vi "Write Name.vi"(8 "error in (no error)":errorcluster, 10 "Name":string, 11 "Config in":refnum<class "Config.lvclass">) -> (0 "error out":errorcluster, 3 "Config out":refnum<class "Config.lvclass">)   [LabVIEW 2018, in "Config.lvclass"]
uses:
  Config.lvclass
  Config.lvclass/Config.ctl
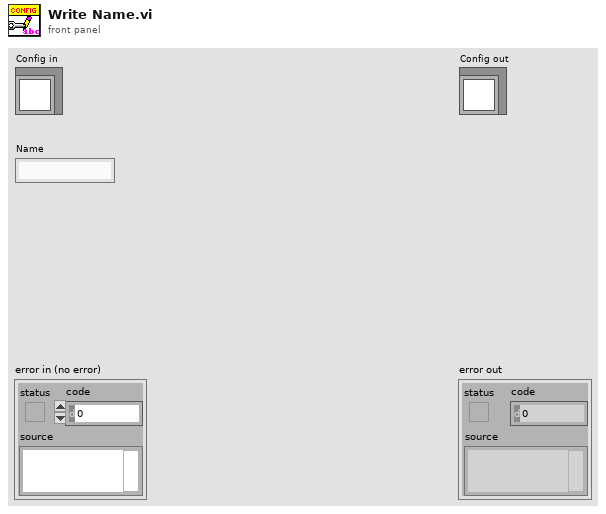
[diagram p1: front panel]
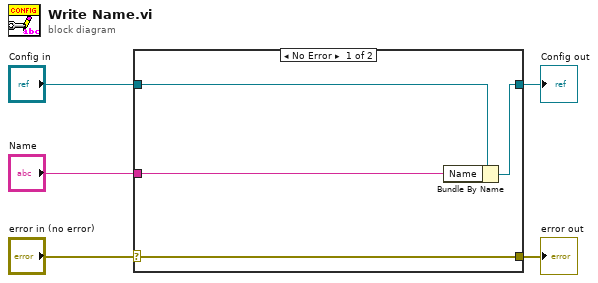
[diagram p0: block diagram]
diagram:
  n1 = case shown="No Error" "error in (no error)" {
    selector: "error in (no error)" -> [w9 w10]
    tunnel: [w9 w10] -> w4
    tunnel: [w7 w11] -> w2
    tunnel: "Config in" -> [w8 w11]
    tunnel: "Name" -> [w6 _]
    frame No Error {
      n2 = Bundle By Name(cluster=w8, "Name"=w6) -> (w7:refnum<class "Config.lvclass">)
    }
    frame Error {
    }
  }
  "error out" <- w4
  "Config out" <- w2
